vi "Select Arguments.vi"(10 "Output Args":refnum<class "Values.lvclass">, 11 "Input Args":refnum<class "Values.lvclass">) -> (3 "Arguments":refnum<class "Values.lvclass">)   [LabVIEW 2020, in "HTTP Server.lvlib" / "Server.lvclass"]
uses:
  Server.lvclass
  Values/Values.lvclass
  Server.lvclass/Server.ctl
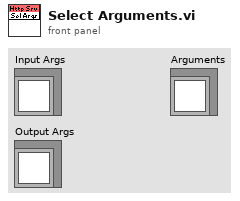
[diagram p1: front panel]
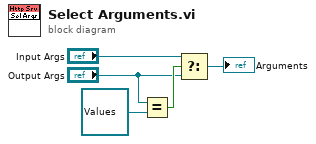
[diagram p0: block diagram]
diagram:
  n1 = Equal?(x="Output Args", y=refnum<class "Values.lvclass"> refnum) -> (x = y?=w4:bool)
  n2 = Select(t="Input Args", s=w4, f="Output Args") -> (s? t:f=→"Arguments":refnum<class "Values.lvclass">)
